vi "Reject Client.vi"(6 "Client":refnum<k5>, 8 "error in (no error)":errorcluster, 11 "Messaging Server Module in":refnum<class "Messaging Server Module.lvclass">) -> (0 "error out":errorcluster, 3 "Messaging Server Module out":refnum<class "Messaging Server Module.lvclass">)   [LabVIEW 2020, in "Volatus.lvlib" / "Messaging Server Module.lvclass"]
uses:
  Messaging Server Module.lvclass
  Messaging Server Module.lvclass/Messaging Server Module.ctl
  lv-vecto/Vecto/proto/ConnectStatus/Enumeration.ctl
  lv-vecto/Vecto/proto/ConnectStatus/ConnectStatus.lvlib
  lv-vecto/Vecto/proto/TcpServerHello/Data.ctl
  lv-vecto/Vecto/proto/TcpServerHello/TcpServerHello.lvlib
  Volatus.lvlib
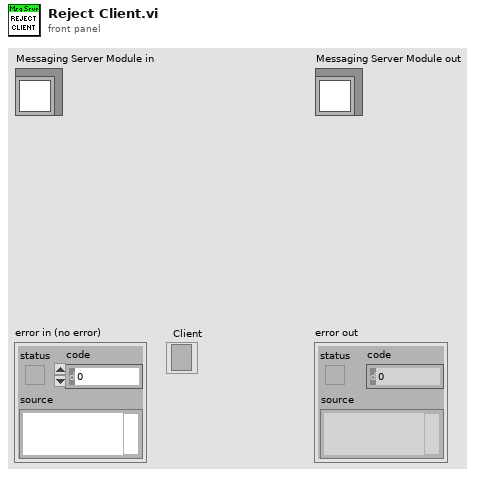
[diagram p1: front panel]
types:
  T1 = typedef "TcpServerHello.lvlib/Data.ctl" = cluster{"status":T2}
  T2 = typedef "ConnectStatus.lvlib/Enumeration.ctl" = enum16{"STATUS_UNKNOWN", "STATUS_SUCCESS", "STATUS_ERROR", "STATUS_BAD_CONFIG", "STATUS_BAD_SYSTEM", "STATUS_BAD_CLUSTER", "STATUS_NOT_ALLOWED"}
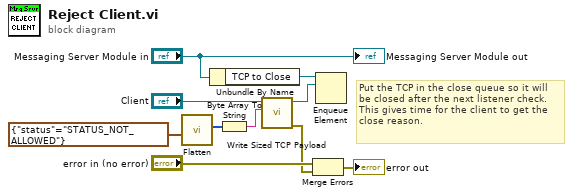
[diagram p0: block diagram]
diagram:
  # "Put the TCP in the close queue so it will be closed after the next listener check. This gives time for the client to get the close reason."
  n1 = call "Flatten.vi"("Data"=T1 {"status"=enum."STATUS_NOT_ALLOWED"} ("TcpServerHello")) -> ("Buffer"=w8:u8[])  [unwired: 9 in, 1 out]
  n2 = Unbundle By Name("Messaging Server Module in") -> ("TCP to Close"=w4:refnum<queue>)
  n3 = Byte Array To String(unsigned byte array=w8) -> (string=w6:string)
  n4 = call "Write Sized TCP Payload.vi"("Payload"=w6, "TCP in"="Client") -> ("error out"=w1:errorcluster, "TCP"=w3:refnum<k5>)  [unwired: 8 in]
  n5 = Merge Errors("error in (no error)", w1) -> (→"error out":errorcluster)
  n6 = Enqueue Element(queue=w4, element=w3) -> ()  [unwired: 2 in, 3 out]
  "Messaging Server Module out" <- "Messaging Server Module in"
